vi "ProcessCompletionWaiterWithOutPut (SubVI).vi"(11 "VISA Refnum in":refnum<visa-resource-name>) -> (3 "Boolean":bool)   [LabVIEW 2020]
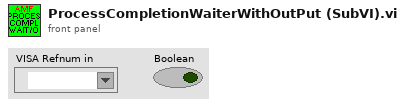
[diagram p1: front panel]
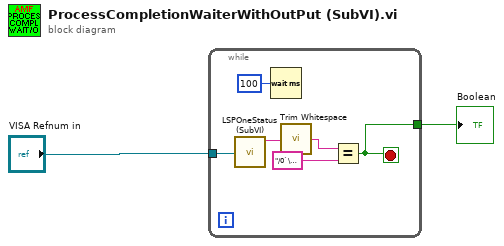
[diagram p0: block diagram]
diagram:
  n1 = while {
    tunnel: "VISA Refnum in" -> [w8]
    tunnel: [w3] -> w2
    stop <- w3 stop-if-true
    n2 = call "LSPOneStatus (SubVI).vi"("VISA Refnum in"=w8) -> ("read buffer"=w6:string)  [unwired: 10 in]
    n3 = Wait (ms)(milliseconds to wait=u32 100) -> ()  [unwired: 1 out]
    n4 = call <vilib>:"Trim Whitespace.vi"("string"=w6) -> ("trimmed string"=w5:string)  [unwired: 1 in]
    n5 = Equal?(x=w5, y="/0`\u0003") -> (x = y?=w3:bool)
  }
  "Boolean" <- w2
